vi "Read String Parameter.vi"(7 "process number":u8, 8 "error in (no error)":errorcluster, 9 "parameter number":u8, 10 "node address (same)":u8, 11 "ProPar in":refnum<class "PL Bronkhorst ProPar.lvclass">) -> (0 "error out":errorcluster, 2 "value":string, 3 "ProPar out":refnum<class "PL Bronkhorst ProPar.lvclass">)   [LabVIEW 2015, in "PL Bronkhorst ProPar.lvclass"]
doc: "Reads specified string <b>parameter</b> of the specified <b>node</b>."
uses:
  PL Bronkhorst ProPar.lvclass
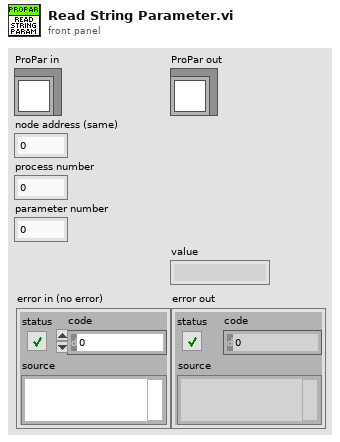
[diagram p1: front panel]
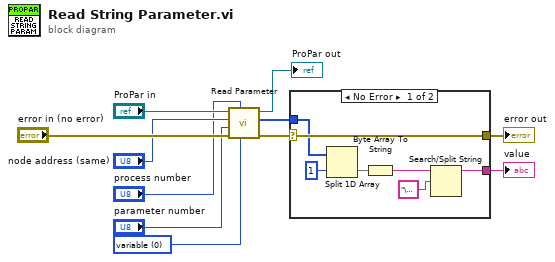
[diagram p0: block diagram]
diagram:
  w1 = u8 0 items=["variable"=0, "1"=1, "2"=2, "4"=4] ("value byte count (variable)")
  n1 = call "Read Parameter.vi"("value byte count"=w1, "process number"="process number", "error in (no error)"="error in (no error)", "parameter number"="parameter number", "node"="node address (same)", "ProPar in"="ProPar in") -> ("error out"=w5:errorcluster, "value"=w4:u8[], "ProPar out"=→"ProPar out":refnum<class "PL Bronkhorst ProPar.lvclass">)  [unwired: 3 in]
  n2 = case shown="No Error" w5 {
    selector: w5 -> [w18 w19]
    tunnel: [w18 w19] -> w2
    tunnel: w4 -> [w17 _]
    tunnel: [w16 _] -> w3
    frame No Error {
      n3 = Split 1D Array(array=w17, index=1) -> (second subarray=w14:u8[])  [unwired: 1 out]
      n4 = Byte Array To String(unsigned byte array=w14) -> (string=w13:string)
      n5 = Search/Split String(string=w13, search string/char (-)="\u0000") -> (substring before match=w16:string)  [unwired: 1 in, 2 out]
    }
    frame Error {
    }
  }
  "error out" <- w2
  "value" <- w3
